vi "Pressure Controller for Module.vi"(8 "error in (no error)":errorcluster) -> (0 "error out":errorcluster)   [LabVIEW 2016]
uses:
  <vilib>/DAQmx/write.llb/DAQmx Write (Digital Bool 1Line 1Point).vi
  <vilib>/DAQmx/create/channels.llb/DAQmx Create Channel (DO-Digital Output).vi
  <vilib>/DAQmx/miscellaneous.llb/DAQmx Fill In Error Info.vi
panel:
  out "Output status of module pressure":bool
  in  "data":bool
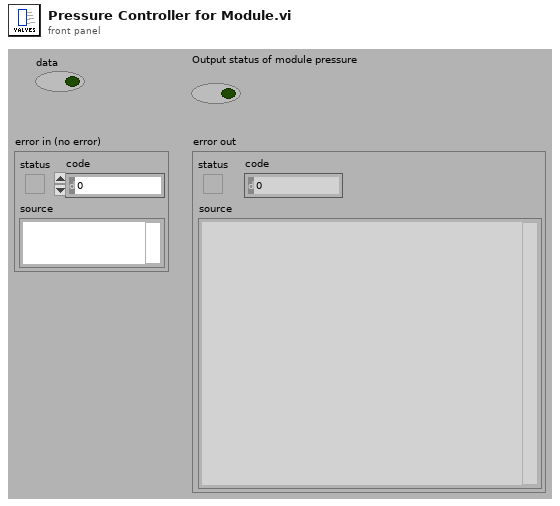
[diagram p1: front panel]
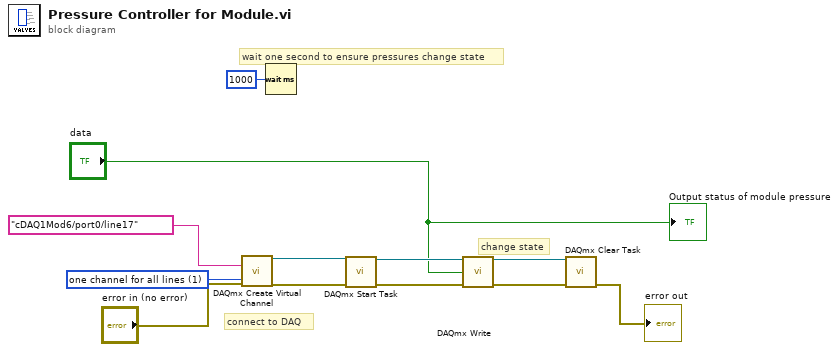
[diagram p0: block diagram]
diagram:
  w11 = 1 items=["one channel for each line", "one channel for all lines"] ("line grouping")
  # "change state"
  # "connect to DAQ"
  # "wait one second to ensure pressures change state"
  n1 = call-poly <vilib>:"DAQmx Create Virtual Channel.vi"("lines"=tag "cDAQ1Mod6/port0/line17" ("Lines"), "line grouping"=w11, "error in"="error in (no error)") -> ("task out"=w9:refnum<k21>, "error out"=w8:errorcluster)  [unwired: 2 in, 9 out]
  n2 = Wait (ms)(milliseconds to wait=u32 1000) -> ()  [unwired: 1 out]
  n3 = call <vilib>:"DAQmx Start Task.vi"("task/channels in"=w9, "error in"=w8) -> ("task out"=w7:refnum<k21>, "error out"=w6:errorcluster)  [unwired: 12 out]
  n4 = call-poly <vilib>:"DAQmx Write.vi"("task/channels in"=w7, "data"="data", "error in"=w6) -> ("task out"=w5:refnum<k21>, "error out"=w4:errorcluster)  [unwired: 1 in, 10 out]
  n5 = call <vilib>:"DAQmx Clear Task.vi"("task in"=w5, "error in"=w4) -> ("error out"=→"error out":errorcluster)  [unwired: 13 out]
  "Output status of module pressure" <- "data"
